vi "Natt Sequence.vi"   [LabVIEW 2020]
uses:
  0b9e1ba2-9ae8-46c0-856f-7726ab11ee73.vi
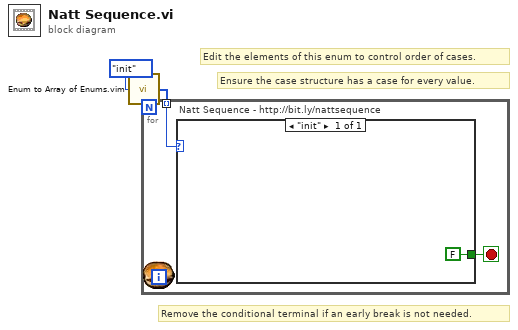
[diagram p0: block diagram]
diagram:
  # "Remove the conditional terminal if an early break is not needed."
  # "Ensure the case structure has a case for every value."
  # "Edit the elements of this enum to control order of cases."
  n1 = call "Enum to Array of Enums.vim"("enum"=enum16{"init"}."init") -> ("array of enums"=w1:enum16{"init"}[])
  n2 = for {
    tunnel: w1 -> [w4] mode=indexing
    stop <- w3 stop-if-true
    # "Natt Sequence - http://bit.ly/nattsequence"
    n3 = case shown="\"init\"" w4 {
      tunnel: [FALSE] -> w3
      frame "init" {
      }
    }
  }
